vi "计算数据合并.vi"(1 "特征点坐标":dbl[](array[numeric]), 2 "声参数":dbl[](array[numeric]), 3 "精度":i16=2, 4 "当前组":dbl format="%#_13g") -> (0 "合并数组":string[][](array[string]))   [LabVIEW 2014]
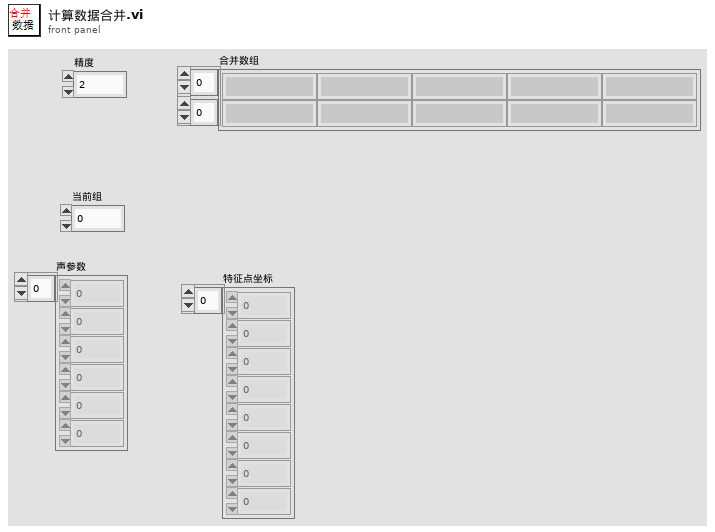
[diagram p1: front panel]
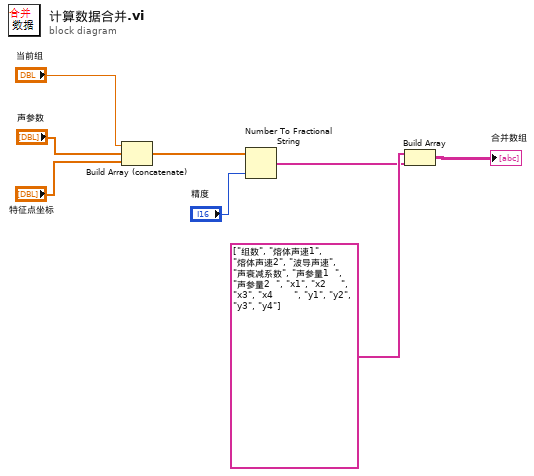
[diagram p0: block diagram]
diagram:
  n1 = Build Array (concatenate)("当前组", "声参数", "特征点坐标") -> (w3:dbl[])
  n2 = Number To Fractional String(number=w3, precision (6)="精度") -> (F-format string=w1:string[])  [unwired: 2 in]
  n3 = Build Array(string[] ["组数", "熔体声速1", "熔体声速2", "波导声速", "声衰减系数", "声参量1  ", "声参量2  ", "x1", "x2     ", "x3", "x4       ", "y1", "y2", "y3", "y4"] ("新元素/子数组"), w1) -> (→"合并数组":string[][])
